vi "File_data_cineticaS1.vi"(8 "path in":path=path "C:/H2_Painel/painel_auto/00100_cinetica.txt", 9 "Nota 01":string, 10 "Sample name":string, 11 "File name":string) -> (0 "path":path)   [LabVIEW 2011]
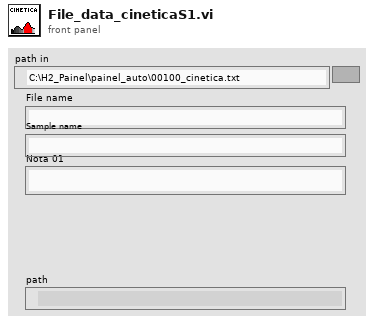
[diagram p1: front panel]
types:
  T1 = enum16{"open", "replace", "create", "open or create", "replace or create", "replace or create with confirmation"}
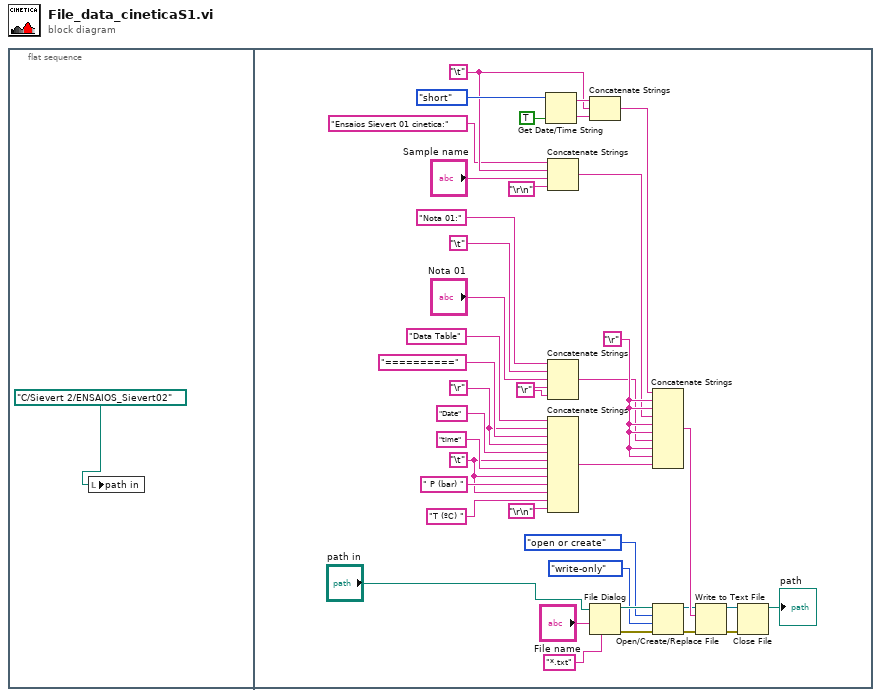
[diagram p0: block diagram]
diagram:
  n1 = flat-sequence {
    frame #0 {
      n2 = local write "path in"(path "C:/Sievert 2/ENSAIOS_Sievert02" ("path in 2")) -> ()
    }
    frame #1 {
      w6 = "\t"
      w5 = "\r"
      w27 = "\r"
      w24 = "\r"
      w9 = "\t"
      n3 = Get Date/Time String(date format (0)=enum16{"short", "long", "abbreviated"}."short", want seconds? (F)=TRUE) -> (date string=w36:string, time string=w35:string)  [unwired: 1 in]
      n4 = Concatenate Strings("Ensaios Sievert 01 cinetica:" ("string"), w9, "Sample name", "\r\n") -> (w7:string)
      n5 = Concatenate Strings("Nota 01:" ("Nota 4"), "\t", "Nota 01", w5, w5) -> (w22:string)
      n6 = Concatenate Strings("Data Table" ("string"), w27, "==========" ("string"), w27, "Date" ("string"), w6, "time" ("string"), w6, " P (bar) " ("string"), w6, "T (ºC) " ("string"), "\r\n") -> (w25:string)
      n7 = Concatenate Strings(w36, w9, w35) -> (w26:string)
      n8 = File Dialog(6:"*.txt" ("pattern label"), 9:"File name", 11:"path in") -> (0:w20:errorcluster, 3:w21:path)  [unwired: 2 in, 4 out]
      n9 = Concatenate Strings(w26, w24, w24, w7, w24, w24, w22, w24, w24, w25) -> (w34:string)
      n10 = Open/Create/Replace File(file path (use dialog)=w21, error in=w20, operation (0:open)=T1."open or create", access (0:read/write)=enum16{"read/write", "read-only", "write-only"}."write-only") -> (refnum out=w17:refnum<file>, error out=w16:errorcluster)  [unwired: 3 out]
      n11 = Write to Text File(file (use dialog)=w17, text=w34, error in=w16) -> (refnum out=w15:refnum<file>, error out=w12:errorcluster)  [unwired: 1 in, 1 out]
      n12 = Close File(refnum=w15, error in=w12) -> (path=→"path":path)  [unwired: 1 out]
    }
  }
